vi "GetTemperature.vi"(8 "Error In":errorcluster, 11 "Omega CSi32 In":refnum<visa-resource-name>) -> (0 "Error Out":errorcluster, 1 "Connected?":bool, 2 "Temperature (C)":dbl format="%.1f", 3 "Omega CSi32 Out":refnum<visa-resource-name>)   [LabVIEW 2012, in "Omega-CSi32.lvlib"]
uses:
  Omega-CSi32.lvlib
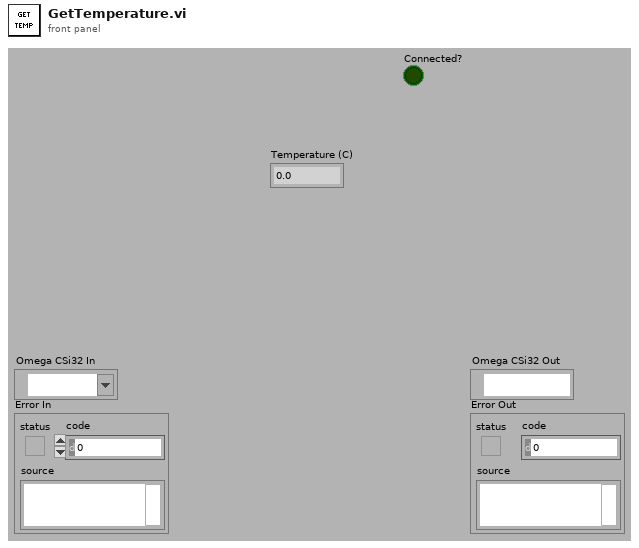
[diagram p1: front panel]
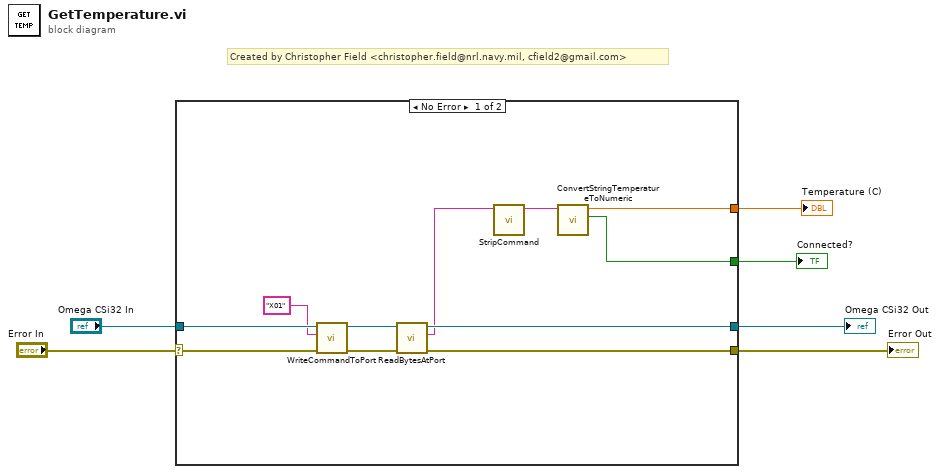
[diagram p0: block diagram]
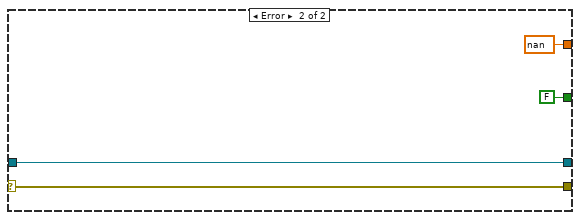
[diagram p2: hidden frame]
diagram:
  # "Created by Christopher Field <christopher.field@nrl.navy.mil, cfield2@gmail.com>"
  n1 = case shown="No Error" "Error In" {
    selector: "Error In" -> [w7 w20]
    tunnel: [w16 nan ("Temperature (C)")] -> w6
    tunnel: [w15 FALSE ("Connected?")] -> w5
    tunnel: "Omega CSi32 In" -> [w14 w21]
    tunnel: [w10 w21] -> w3
    tunnel: [w9 w20] -> w2
    frame No Error {
      n2 = call "WriteCommandToPort.vi"("Error In"=w7, "Command"="X01", "CSi32 In"=w14) -> ("Error Out"=w11:errorcluster, "CSi32 Out"=w12:refnum<visa-resource-name>)  [unwired: 7 in]
      n3 = call "ReadBytesAtPort.vi"("Error In"=w11, "CSi32 In"=w12) -> ("Error Out"=w9:errorcluster, "Read Buffer"=w8:string, "CSi32 Out"=w10:refnum<visa-resource-name>)  [unwired: 7 in]
      n4 = call "StripCommand.vi"("Command"=w8) -> ("Stripped Command"=w17:string)  [unwired: 10 in]
      n5 = call "ConvertStringTemperatureToNumeric.vi"("Temperature"=w17) -> ("Connected?"=w15:bool, "Temperature (C)"=w16:dbl)  [unwired: 9 in]
    }
    frame Error {
    }
  }
  "Omega CSi32 Out" <- w3
  "Error Out" <- w2
  "Temperature (C)" <- w6
  "Connected?" <- w5
